vi "librequest_available.vi"(8 "error in (no error)":errorcluster, 11 "output":i32) -> (0 "error out":errorcluster, 2 "is":bool)   [LabVIEW 2015]
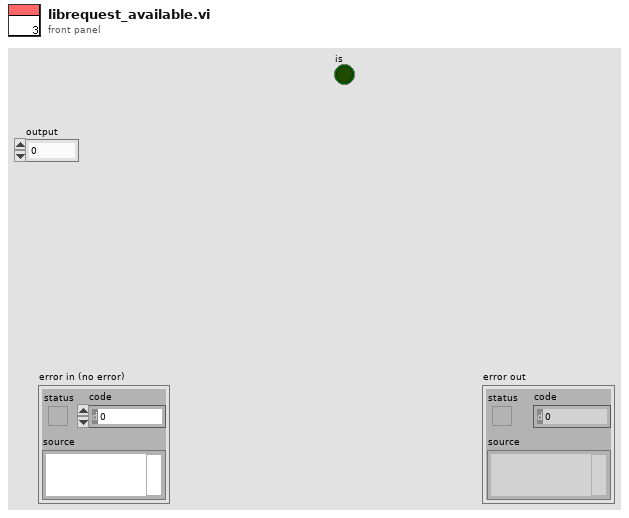
[diagram p1: front panel]
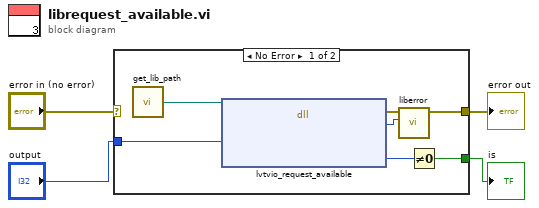
[diagram p0: block diagram]
diagram:
  n1 = case shown="No Error" "error in (no error)" {
    selector: "error in (no error)" -> [_ w12]
    tunnel: [w5 w12] -> w3
    tunnel: [w9 _] -> w2
    tunnel: "output" -> [w8 _]
    frame No Error {
      n2 = call "get_lib_path.vi"() -> ("Path"=w11:path)
      n3 = dll-call lib="S:/thingiverselv/lib/liblvtvio.dll" fn="lvtvio_request_available"(path in=w11, "output"=w8) -> (error out=w6:errorcluster, "return type"=w7:i32, "is"=w10:i32)  [unwired: 4 in, 1 out]
      n4 = call "liberror.vi"("tvio errors"=w7, "error in (no error)"=w6) -> ("error out"=w5:errorcluster)  [unwired: 9 in]
      n5 = Not Equal To 0?(x=w10) -> (x != 0?=w9:bool)
    }
    frame Error {
    }
  }
  "error out" <- w3
  "is" <- w2
